vi "Enumerate_Cameras.vi"(8 "error in (no error)":errorcluster, 11 "Ring in":refnum<vi>) -> (0 "error out":errorcluster, 3 "reference out":refnum<vi>)   [LabVIEW 2023, in "Camera_Controller.lvlib"]
uses:
  Camera_Controller.lvlib
  <vilib>/vision/driver/NI_Vision_Acquisition_Software.lvlib
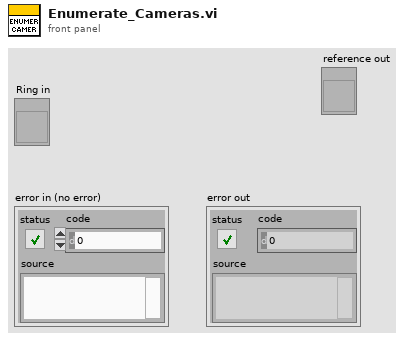
[diagram p1: front panel]
types:
  T1 = cluster{"Type":u32, "Version":u32, "Flags":u32, "SerialNumberHigh":u32, "SerialNumberLow":u32, "BusType":u32, "InterfaceName":string, "VendorName":string, "ModelName":string, "CameraFileName":string, "CameraAttributeURL":string}[]
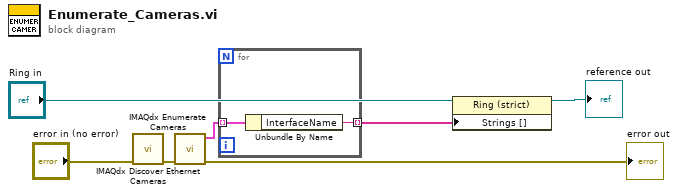
[diagram p0: block diagram]
diagram:
  n1 = call <vilib>:"IMAQdx Discover Ethernet Cameras.vi"("error in"="error in (no error)") -> ("error out"=w4:errorcluster)  [unwired: 10 in]
  n2 = call <vilib>:"IMAQdx Enumerate Cameras.vi"("error in"=w4) -> ("error out"=→"error out":errorcluster, "Camera Information Array"=w3:T1)  [unwired: 9 in]
  n3 = for {
    tunnel: w3 -> [w9] mode=indexing
    tunnel: [w8] -> w2 mode=indexing
    n4 = Unbundle By Name(w9) -> ("InterfaceName"=w8:string)
  }
  n5 = property on="Property Node" class="Ring (strict)"(reference="Ring in", "Strings []"=w2) -> (reference out=→"reference out":refnum<vi>)  [unwired: 1 in, 1 out]
